vi "GET_CONFIGURATION_DATA_n.vi"(5 "error in (no error)":errorcluster, 8 "execute":bool) -> (1 "data":string, 9 "Shunt":string, 10 "BinCnt":u16=15, 11 "CompValues":string, 12 "function return":string, 14 "DFTBins":u16[](array[numeric])=[1, 2, 3, 7, 11, 17, 23, 31, 43, 61, 89, 127, 179, 251, 349], 15 "ShuntImpedanceReal":sgl[](array[numeric])=[1000.0, 1000.0, 1000.0, 1000.0, 1000.0, 1000.0, 1000.0, 1000.0, 1000.0, 1000.0, 1000.0, 1000.0, 1000.0, 1000.0, 1000.0], 16 "ShuntImpedanceImaginary":sgl[](array[numeric]), 17 "InputCompenValReal":sgl[](array[numeric])=[1000000000.0, 1000000000.0, 1000000000.0, 1000000000.0, 1000000000.0, 1000000000.0, 1000000000.0, 1000000000.0, 1000000000.0, 1000000000.0, 1000000000.0, 1000000000.0, 1000000000.0, 1000000000.0, 1000000000.0], 18 "InputCompenValImaginary":sgl[](array[numeric]), 19 "error out":errorcluster)   [LabVIEW 2017, in "ZBOX_IS.lvlib"]
uses:
  ZBOX_IS.lvlib
panel:
  out "length":i32=272
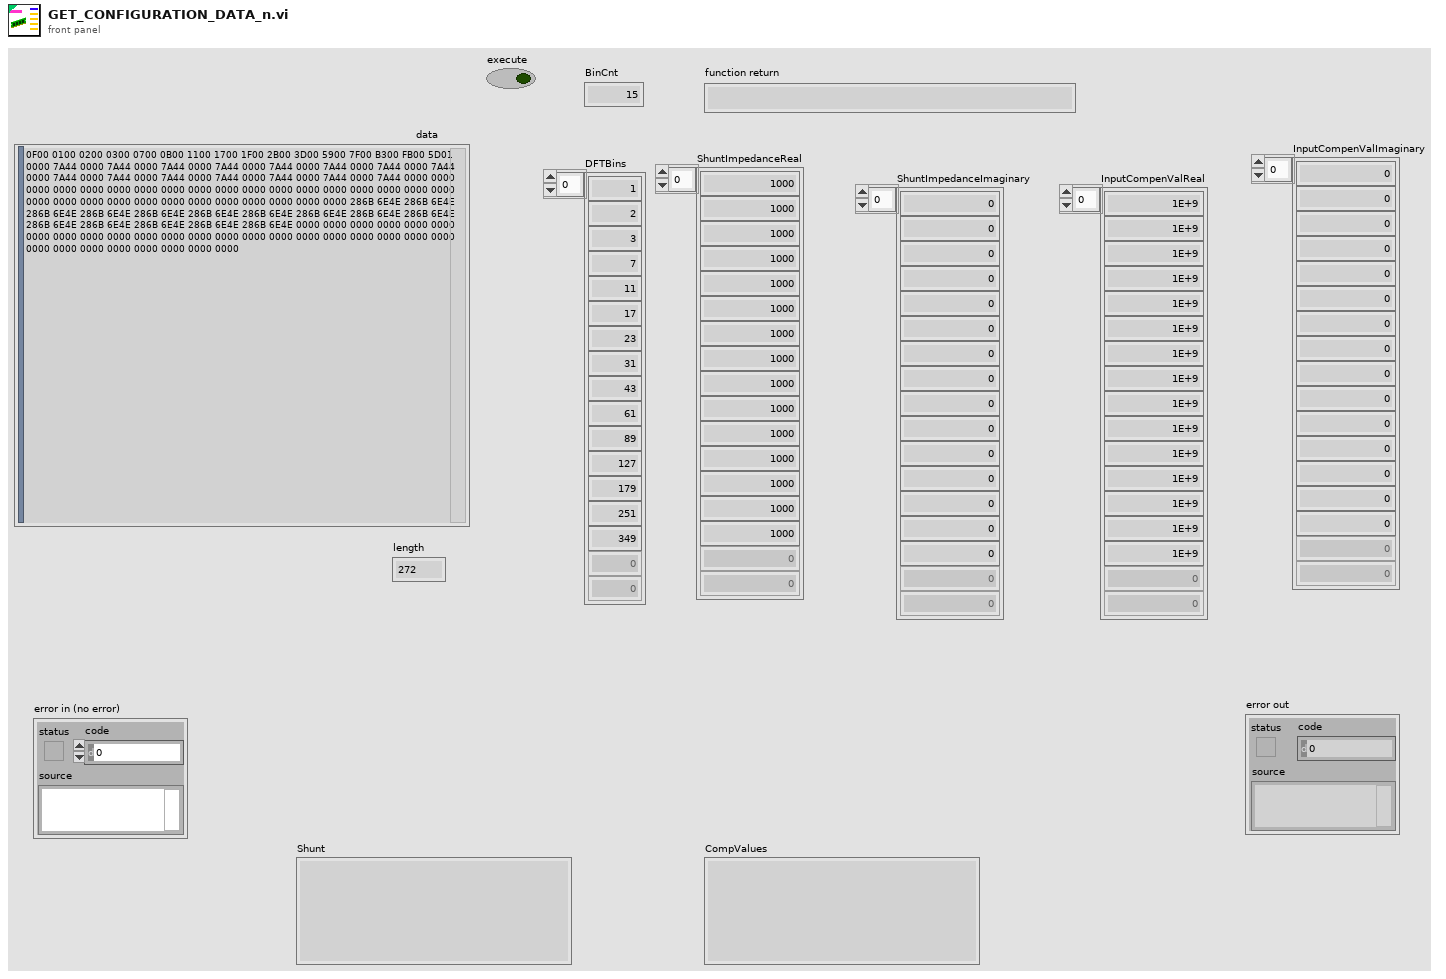
[diagram p1: front panel]
types:
  T1 = enum16{"big-endian, network order", "native, host order", "little-endian"}
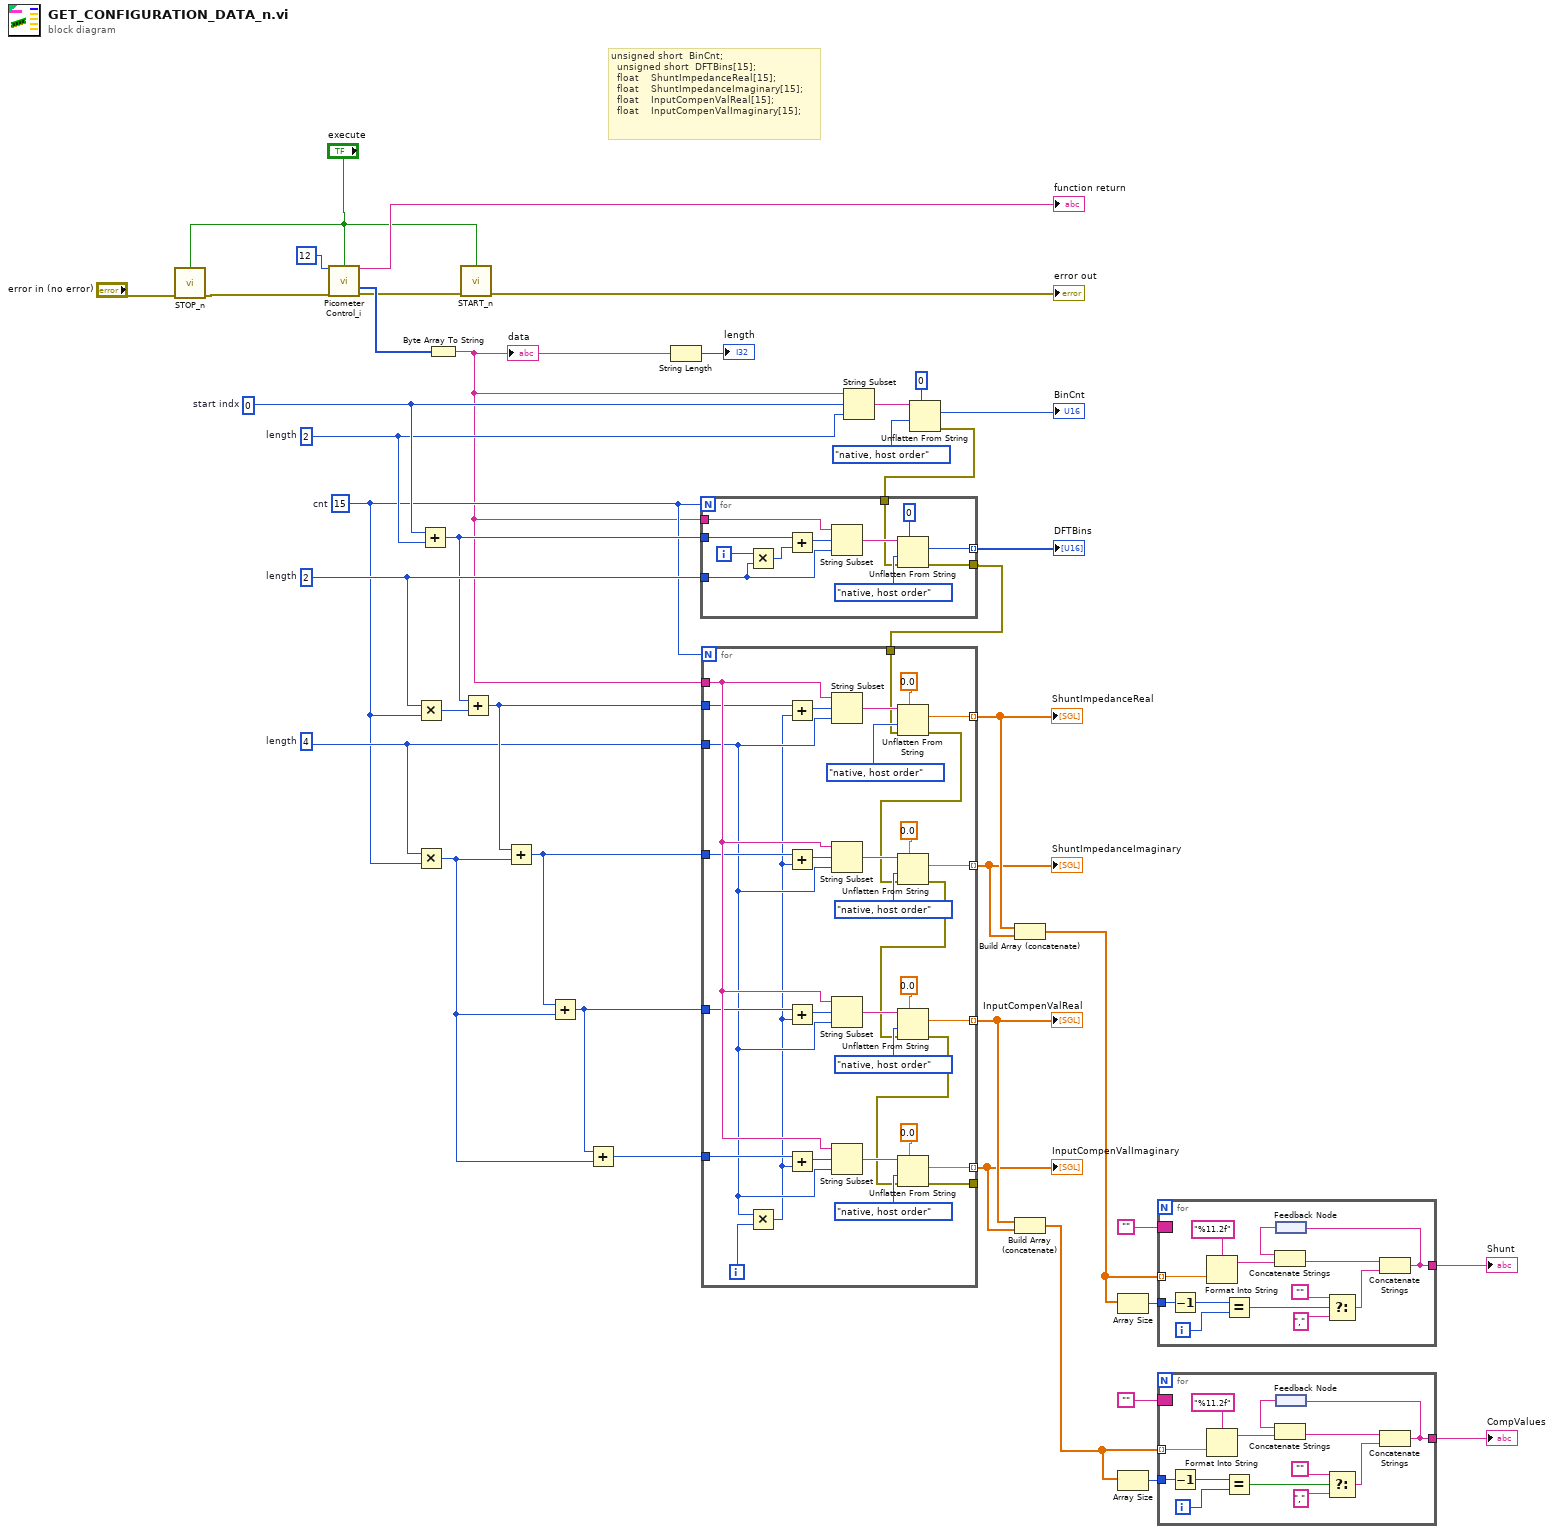
[diagram p0: block diagram]
diagram:
  w26 = 4  # length
  w34 = 2  # length
  w36 = 0  # start indx
  w35 = 2  # length
  w25 = 15  # cnt
  # "unsigned short\t\tBinCnt;\n\t\tunsigned short\t\tDFTBins[15];\n\t\tfloat\t\t\t\tShuntImpedanceReal[15];\n\t\tfloat\t\t\t\tShuntImpedanceImaginary[15];\n\t\tfloat\t\t\t\tInputCompenValReal[15];\n\t\tfloat\t\t\t\tInputCompenValImaginary[15];"
  n1 = call "STOP_n.vi"("execute"="execute", "error in (no error)"="error in (no error)") -> ("error out"=w19:errorcluster)  [unwired: 12 in, 1 out]
  n2 = call "Picometer Control_i.vi"("Cmd"=u8 12, "execute"="execute", "error in (no error)"=w19) -> ("function return"=→"function return":string, "BytePtr"=w23:u8[], "error out"=w18:errorcluster)  [unwired: 8 in, 2 out]
  n3 = Multiply(x=w34, y=w25) -> (x*y=w32:i32)
  n4 = Multiply(x=w26, y=w25) -> (x*y=w28:i32)
  n5 = Add(x=w36, y=w35) -> (x+y=w33:i32)
  n6 = Byte Array To String(unsigned byte array=w23) -> (string=w22:string)
  "data" <- w22
  n7 = call "START_n.vi"("execute"="execute", "error in (no error)"=w18) -> ("error out"=→"error out":errorcluster)  [unwired: 12 in, 1 out]
  n8 = Add(x=w33, y=w32) -> (x+y=w31:i32)
  n9 = Add(x=w31, y=w28) -> (x+y=w30:i32)
  n10 = Add(x=w30, y=w28) -> (x+y=w29:i32)
  n11 = Add(x=w29, y=w28) -> (x+y=w27:i32)
  n12 = String Length(string=w22) -> (length=→"length":i32)
  n13 = String Subset(string=w22, offset (0)=w36, length (rest)=w35) -> (substring=w39:string)
  n14 = Unflatten From String(type=u16 0, binary string=w39, byte order (0:big-endian, network order)=T1."native, host order" ("byte order (0:big-endian, network order) 2")) -> (value=→"BinCnt":u16, error out=w2:errorcluster)  [unwired: 2 in, 1 out]
  n15 = for {
    N: w25 -> [_]
    tunnel: w22 -> [w49]
    tunnel: [w48] -> w4 mode=indexing
    tunnel: w33 -> [w51]
    tunnel: [w47] -> w1
    tunnel: w34 -> [w43]
    tunnel: w2 -> [w42]
    i -> [w53]
    n16 = Multiply(x=w53, y=w43) -> (x*y=w50:i32)
    n17 = Add(x=w51, y=w50) -> (x+y=w52:i32)
    n18 = String Subset(string=w49, offset (0)=w52, length (rest)=w43) -> (substring=w45:string)
    n19 = Unflatten From String(type=u16 0, binary string=w45, byte order (0:big-endian, network order)=T1."native, host order" ("byte order (0:big-endian, network order) 2"), error in (no error)=w42) -> (value=w48:u16, error out=w47:errorcluster)  [unwired: 1 in, 1 out]
  }
  "DFTBins" <- w4
  n20 = for {
    N: w25 -> [_]
    tunnel: [w86] -> w11 mode=indexing
    tunnel: w22 -> [w85]
    tunnel: [w84] -> w13 mode=indexing
    tunnel: [w83] -> w14 mode=indexing
    tunnel: [w82] -> w10 mode=indexing
    tunnel: w31 -> [w81]
    tunnel: w30 -> [w80]
    tunnel: w29 -> [w79]
    tunnel: w27 -> [w78]
    tunnel: w26 -> [w76]
    tunnel: [w71] -> _
    tunnel: w1 -> [w57]
    i -> [w77]
    n21 = Multiply(x=w76, y=w77) -> (x*y=w58:i32)
    n22 = Add(x=w81, y=w58) -> (x+y=w62:i32)
    n23 = Add(x=w80, y=w58) -> (x+y=w66:i32)
    n24 = Add(x=w79, y=w58) -> (x+y=w70:i32)
    n25 = Add(x=w78, y=w58) -> (x+y=w75:i32)
    n26 = String Subset(string=w85, offset (0)=w62, length (rest)=w76) -> (substring=w61:string)
    n27 = String Subset(string=w85, offset (0)=w66, length (rest)=w76) -> (substring=w65:string)
    n28 = String Subset(string=w85, offset (0)=w70, length (rest)=w76) -> (substring=w69:string)
    n29 = String Subset(string=w85, offset (0)=w75, length (rest)=w76) -> (substring=w74:string)
    n30 = Unflatten From String(type=sgl 0.0, binary string=w61, byte order (0:big-endian, network order)=T1."native, host order" ("byte order (0:big-endian, network order) 2"), error in (no error)=w57) -> (value=w86:sgl, error out=w56:errorcluster)  [unwired: 1 in, 1 out]
    n31 = Unflatten From String(type=sgl 0.0, binary string=w65, byte order (0:big-endian, network order)=T1."native, host order" ("byte order (0:big-endian, network order) 2"), error in (no error)=w56) -> (value=w82:sgl, error out=w55:errorcluster)  [unwired: 1 in, 1 out]
    n32 = Unflatten From String(type=sgl 0.0, binary string=w69, byte order (0:big-endian, network order)=T1."native, host order" ("byte order (0:big-endian, network order) 2"), error in (no error)=w55) -> (value=w83:sgl, error out=w54:errorcluster)  [unwired: 1 in, 1 out]
    n33 = Unflatten From String(type=sgl 0.0, binary string=w74, byte order (0:big-endian, network order)=T1."native, host order" ("byte order (0:big-endian, network order) 2"), error in (no error)=w54) -> (value=w84:sgl, error out=w71:errorcluster)  [unwired: 1 in, 1 out]
  }
  "ShuntImpedanceReal" <- w11
  "ShuntImpedanceImaginary" <- w10
  "InputCompenValReal" <- w14
  "InputCompenValImaginary" <- w13
  n34 = Build Array (concatenate)(w11, w10) -> (w7:sgl[])
  n35 = Build Array (concatenate)(w14, w13) -> (w12:sgl[])
  n36 = Array Size(array=w7) -> (size(s)=w8:i32)
  n37 = Array Size(array=w12) -> (size(s)=w16:i32)
  n38 = for {
    tunnel: w7 -> [w99] mode=indexing
    border: "" -> [_]
    tunnel: [w94] -> w5
    tunnel: w8 -> [w93]
    i -> [w92]
    n39 = Decrement(x=w93) -> (x-1=w87:i32)
    n40 = Format Into String(format string="%11.2f", w99) -> (resulting string=w98:string)  [unwired: 2 in, 1 out]
    n41 = Equal?(x=w87, y=w92) -> (x = y?=w90:bool)
    n42 = feedback #1() -> (w97:string)
    n43 = Concatenate Strings(w97, w98) -> (w95:string)
    n44 = Select(t="", s=w90, f="," ("string")) -> (s? t:f=w89:string)
    n45 = Concatenate Strings(w95, w89) -> (w94:string)
    n46 = feedback-in #1(w94) -> ()
  }
  "Shunt" <- w5
  n47 = for {
    tunnel: w12 -> [w112] mode=indexing
    border: "" -> [_]
    tunnel: [w107] -> w6
    tunnel: w16 -> [w106]
    i -> [w105]
    n48 = Decrement(x=w106) -> (x-1=w100:i32)
    n49 = Format Into String(format string="%11.2f", w112) -> (resulting string=w111:string)  [unwired: 2 in, 1 out]
    n50 = Equal?(x=w100, y=w105) -> (x = y?=w103:bool)
    n51 = feedback #2() -> (w110:string)
    n52 = Concatenate Strings(w110, w111) -> (w108:string)
    n53 = Select(t="", s=w103, f="," ("string")) -> (s? t:f=w102:string)
    n54 = Concatenate Strings(w108, w102) -> (w107:string)
    n55 = feedback-in #2(w107) -> ()
  }
  "CompValues" <- w6
